vi "Decode packed enum.vi"(10 "Wire Type":T1, 11 "Data":u8[](array[numeric]) format="%.0x") -> (2 "error out":errorcluster, 3 "Enumeration":T2[](array[typedef]))   [LabVIEW 2020, in "EventLevel.lvlib"]
uses:
  EventLevel.lvlib
  Enumeration.ctl
  lv-protoc/LV-Proto/Wire Type.ctl
  lv-protoc/LV-Proto/LV-Proto.lvlib
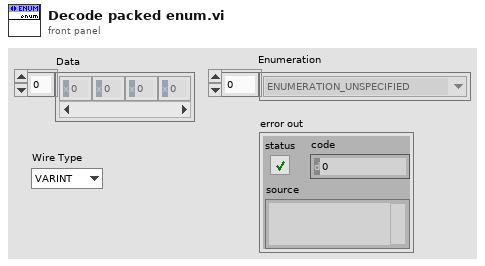
[diagram p1: front panel]
types:
  T1 = typedef "LV-Proto.lvlib/Wire Type.ctl" = enum8{"VARINT", "I64", "LEN", "SGROUP (Deprecated)", "EGROUP (Deprecated)", "I32"}
  T2 = typedef "EventLevel.lvlib/Enumeration.ctl" = enum16{"ENUMERATION_UNSPECIFIED"}
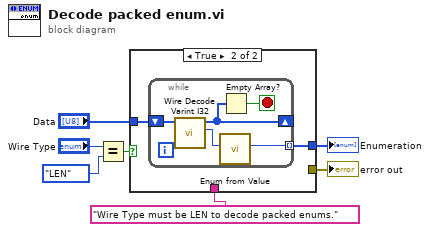
[diagram p0: block diagram]
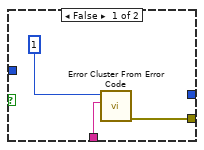
[diagram p2: hidden frame]
diagram:
  n1 = Equal?(x="Wire Type", y=Wire_Type."LEN") -> (x = y?=w7:bool)
  n2 = case shown="True" w7 {
    tunnel: "Data" -> [_ w12]
    tunnel: [w9 _] -> w1
    tunnel: "Wire Type must be LEN to decode packed enums." -> [w8 _]
    tunnel: [_ w11] -> w2
    frame False {
      n3 = call <vilib>:"Error Cluster From Error Code.vi"("error message (\"\")"=w8, "error code (0)"=1) -> ("error out"=w9:errorcluster)  [unwired: 7 in]
    }
    frame True {
      n4 = while {
        tunnel: [w15] -> w11 mode=indexing
        shift-right: [w14] -> _
        shift-left: w12 -> [w17]
        stop <- w13 stop-if-true
        n5 = call "Wire Decode Varint I32.vi"("Buffer in"=w17) -> ("I32"=w16:i32, "Buffer"=w14:u8[])  [unwired: 9 in]
        n6 = call "Enum from Value.vi"("Value"=w16) -> ("Enumeration"=w15:T2)  [unwired: 10 in]
        n7 = Empty Array?(array=w14) -> (empty?=w13:bool)
      }
    }
  }
  "Enumeration" <- w2
  "error out" <- w1
